vi "mqttCmdPublishValueRead.vi"(0 "mqttPublish in":refnum<class "mqttCmdPublish.lvclass">, 11 "error in (no error)":errorcluster) -> (4 "mqttPublish out":refnum<class "mqttCmdPublish.lvclass">, 6 "value":string, 15 "error out":errorcluster)   [LabVIEW 2022 SP3, in "mqttCmdPublish.lvclass"]
uses:
  mqttCmdPublish.lvclass
  mqttCmdPublish.lvclass/mqttCmdPublish.ctl
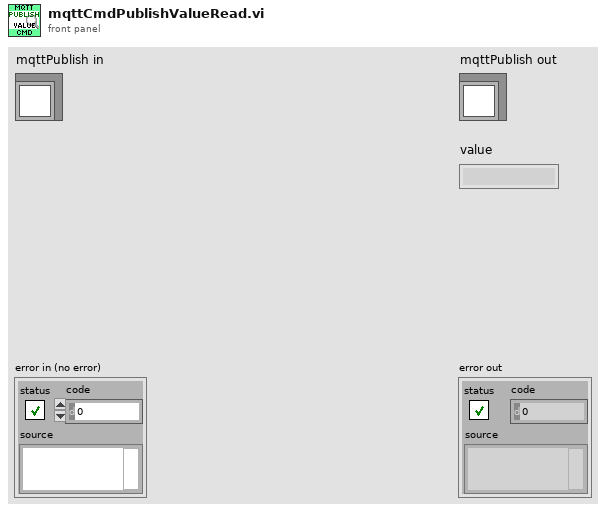
[diagram p1: front panel]
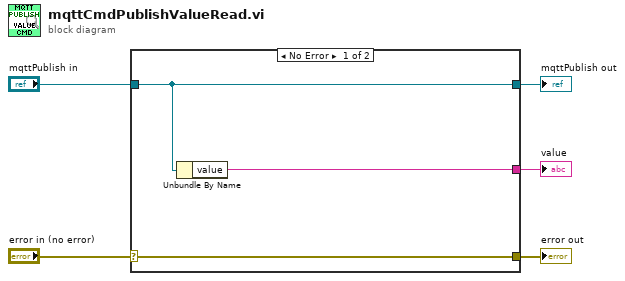
[diagram p0: block diagram]
diagram:
  n1 = case shown="No Error" "error in (no error)" {
    selector: "error in (no error)" -> [w8 w9]
    tunnel: [w8 w9] -> w4
    tunnel: [w7 w10] -> w2
    tunnel: "mqttPublish in" -> [w7 w10]
    tunnel: [w6 _] -> w1
    frame No Error {
      n2 = Unbundle By Name(w7) -> ("value"=w6:string)
    }
    frame Error {
    }
  }
  "error out" <- w4
  "mqttPublish out" <- w2
  "value" <- w1
